vi "Initialize pretomo IMAQ.vi"(8 "error in (no error)":errorcluster, 11 "Tomo in":refnum<class "Tomo.lvclass">) -> (0 "error out":errorcluster, 3 "Tomo out":refnum<class "Tomo.lvclass">)   [LabVIEW 2012, in "Tomo.lvclass"]
uses:
  Tomo.lvclass
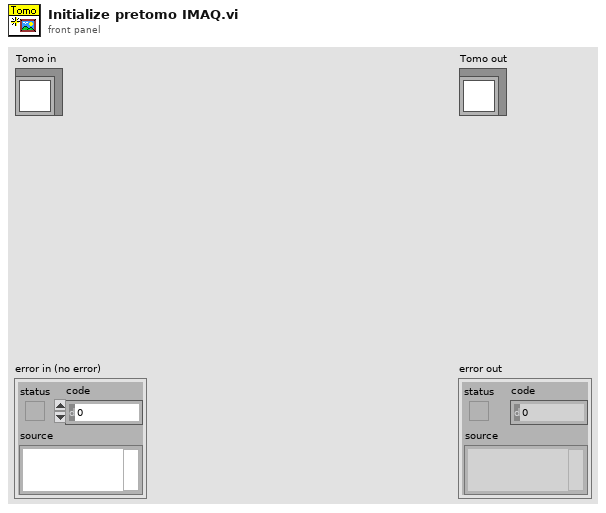
[diagram p1: front panel]
types:
  T1 = typedef "Image Type" = u32
  T2 = typedef "IMAQ Image.ctl" = refnum<image>
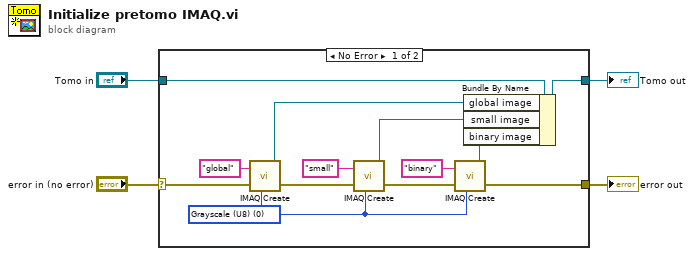
[diagram p0: block diagram]
diagram:
  n1 = case shown="No Error" "error in (no error)" {
    selector: "error in (no error)" -> [w15 w19]
    tunnel: [w14 w19] -> w3
    tunnel: [w11 w18] -> w1
    tunnel: "Tomo in" -> [w12 w18]
    frame No Error {
      w13 = T1 0 items=["Grayscale (U8)", "Grayscale (I16)", "Grayscale (SGL)", "Complex (CSG)", "RGB (U32)", "HSL (U32)", "RGB (U64)", "Grayscale (U16)"] ("Image Type")
      n2 = call "IMAQ Create"("Image Name"="global", "Image Type"=w13, "error in (no error)"=w15) -> ("New Image"=w7:T2, "error out"=w17:errorcluster)  [unwired: 2 in]
      n3 = call "IMAQ Create"("Image Name"="small", "Image Type"=w13, "error in (no error)"=w17) -> ("New Image"=w6:T2, "error out"=w16:errorcluster)  [unwired: 2 in]
      n4 = call "IMAQ Create"("Image Name"="binary", "Image Type"=w13, "error in (no error)"=w16) -> ("New Image"=w5:T2, "error out"=w14:errorcluster)  [unwired: 2 in]
      n5 = Bundle By Name(cluster=w12, "global image"=w7, "small image"=w6, "binary image"=w5) -> (w11:refnum<class "Tomo.lvclass">)
    }
    frame Error {
    }
  }
  "error out" <- w3
  "Tomo out" <- w1
